vi "PH_Sixpack.panel.vi"(0 "object ref":refnum<vi>, 5 "error in (no error)":errorcluster) -> (19 "error out":errorcluster)   [LabVIEW 2014, in "PH_Sixpack.lvlib"]
doc: "By this VI a hardware switch can be monitored and switched. \n\nThe indicators \"FALSE\", \"TRUE\" and \"SWITCH STATE\" show the value of the Beckhoff-Tag: blue indicates bad tag status reference problems, darkgreen false and lightgreen true. If everything is working fine, \"FALSE\" and \"SWITCH STATE\" should show the same value, while \"TRUE\" has the opposite value. The caption of the sensors for \"FALSE\" and \"TRUE\" are taken out of the database. In case of only one or no sensor these GUI elements are not shown at all.\n\nThe oval button switches. It should be in the same state as the \"SWITCH STATE\" indicator. \n\n\"Delete Instance\" disconnects and removes the instance from the PCS.\n\n\nLicense Agreement for this software:\n\nCopyright (C)\nGesellschaft für Schwerionenforschung, GSI\nPlanckstr. 1\n64291 Darmstadt\nGermany\n\nContact: D.Beck@gsi.de \n\nThis program is free software; you can redistribute it and/or modify it under the terms of the GNU General Public License as published by the Free Software Foundation; either version 2 of the license, or (at your option) any later version.\n\nThis program is distributed in the hope that it will be useful, but WITHOUT ANYW ARRANTY; without even the implied warranty of MERCHANTABILITY or FITNESS FOR A PARTICULAR PURPOSE. See the GNU General License for more details (http://www.gnu.org).\n\nGesellschaft für Schwerionenforschung, GSI\nPlanckstr. 1, 64291 Darmstadt, Germany\nFor all questions and ideas contact: M.Richter@gsi.de, H.Brand@gsi.de or D.Beck@gsi.de.\nLast update: 18-DEC-2002"
uses:
  PH_Sixpack.lvlib
  PH_Stepmotor_BaseClass/PH_Stepmotor_BaseClass.Axis Settings.ctl
  PH_Stepmotor_BaseClass/PH_Stepmotor_BaseClass.Motor Type.ctl
  PH_Stepmotor_BaseClass/PH_Stepmotor_BaseClass.Axis Information.ctl
  PH_Stepmotor_BaseClass/PH_Stepmotor_BaseClass.Axis Activity.ctl
  PH_Sixpack.Status.ctl
  PH_Sixpack.Axis Cluster.ctl
  PH_Sixpack.Axis Configuration.ctl
  instr.lib/SixPack/PackDLL/VmaxAmax.ctl
  instr.lib/SixPack/PackDLL/PeakCurrent.ctl
  instr.lib/SixPack/PackDLL/VStartVmin.ctl
  instr.lib/SixPack/PackDLL/Ref Search Parameter.ctl
  instr.lib/SixPack/PackDLL/Stopswitch Limits.ctl
  instr.lib/SixPack/PackDLL/Motor Parameter.ctl
  instr.lib/SixPack/PackDLL/MotorParameter_P5.ctl
  instr.lib/SixPack/PackDLL/MotorParameter_P6.ctl
  instr.lib/SixPack/PackDLL/Current Control.ctl
  instr.lib/SixPack/PackDLL/Current.ctl
  PH_Sixpack.Input.ctl
  PH_Stepmotor_BaseClass/PH_Stepmotor_BaseClass.GUI Refs.ctl
  CSCore/CSObj/CSObj.lvlib
  PH_Common/PH_Common.lvlib
  PH_Stepmotor_BaseClass/PH_Stepmotor_BaseClass.lvlib
  PH_Class/PH_Class.lvlib
  instr.lib/SixPack/Sixpack - Driver.lvlib
panel:
  out "PeriodicInterval [ms]":i32=-1
  out "Inputs":T1[](array[typedef])
  out "Axes Configuration (Sixpack)":T2[](array[typedef]) {"Config"."Axis Parameter"."Poslimit (6400)" step=1; "Config"."Ref Search Parameter"."DebouncingTime (22ms)" format="%.0x"; "Config"."I max (50%)" min=0.0 max=100.0}
  out "Axes PSDB Infos":T14(array[cluster])
  out "Axis to do a RefSearch":i32=-1
  out "Status":T15
  out "Firmwareversion":dbl=-1.0
  out "Serial Number":dbl=-1.0
  out "Information":T16={"SixPack ID(0)"=0, "BaudRate(19200)"=19200, "COM Port"=enum."COM1", "HANDLE"=0}
  out "Device Error":errorcluster
  out "Axes Configuration (Base Class)":T21(array[cluster])
  in  "Stop":bool caption="SetZero"
  out "PSDB Status":u32(colorbox)=6618880 caption="PSDB"
  in  "Exit":bool
  in  "Delete":bool
  # "PCS"
  # "3.40"
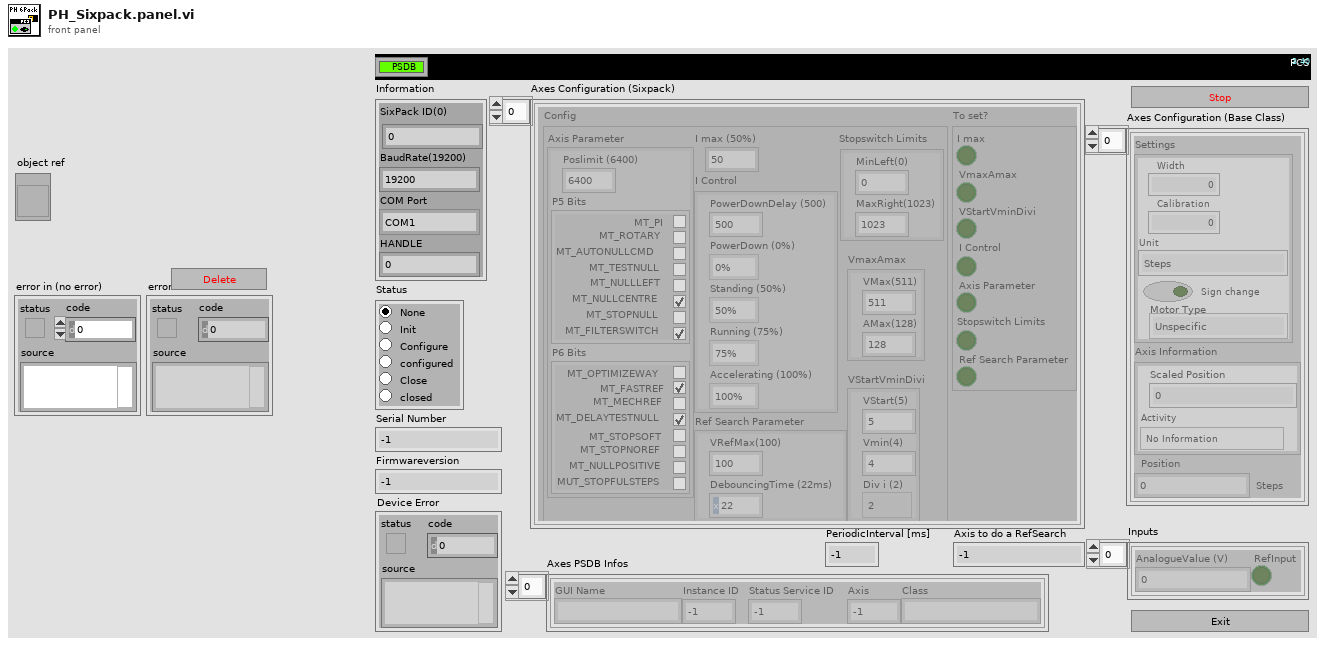
[diagram p1: front panel]
types:
  T1 = typedef "PH_Sixpack.lvlib/PH_Sixpack.Input.ctl" = cluster{"AnalogueValue (V)":dbl, "RefInput":bool}
  T2 = typedef "PH_Sixpack.lvlib/PH_Sixpack.Axis Cluster.ctl" = cluster{"Config":T3, "To set?":cluster{"VmaxAmax":bool, "I max":bool, "VStartVminDivi":bool, "Ref Search Parameter":bool, "Stopswitch Limits":bool, "Axis Parameter":bool, "I Control":bool}}
  T3 = typedef "PH_Sixpack.lvlib/PH_Sixpack.Axis Configuration.ctl" = cluster{"VmaxAmax":T4, "I max (50%)":T5, "VStartVminDivi":T6, "Ref Search Parameter":T7, "Stopswitch Limits":T8, "Axis Parameter":T9, "I Control":T12}
  T4 = typedef "Sixpack - Driver.lvlib/VmaxAmax.ctl" = cluster{"VMax(511)":u16, "AMax(128)":u16}
  T5 = typedef "Sixpack - Driver.lvlib/PeakCurrent.ctl" = dbl
  T6 = typedef "Sixpack - Driver.lvlib/VStartVmin.ctl" = cluster{"VStart(5)":u16, "Vmin(4)":u16, "Div i (2)":enum8{"0", "1", "2", "3"}}
  T7 = typedef "Sixpack - Driver.lvlib/Ref Search Parameter.ctl" = cluster{"VRefMax(100)":u16, "DebouncingTime (22ms)":u8}
  T8 = typedef "Sixpack - Driver.lvlib/Stopswitch Limits.ctl" = cluster{"MinLeft(0)":u16, "MaxRight(1023)":u16}
  T9 = typedef "Sixpack - Driver.lvlib/Motor Parameter.ctl" = cluster{"Poslimit (6400)":u32, "P5 Bits":T10, "P6 Bits":T11}
  T10 = typedef "Sixpack - Driver.lvlib/MotorParameter_P5.ctl" = cluster{"MT_PI":bool, "MT_ROTARY":bool, "MT_AUTONULLCMD":bool, "MT_TESTNULL":bool, "MT_NULLLEFT":bool, "MT_NULLCENTRE":bool, "MT_STOPNULL":bool, "MT_FILTERSWITCH":bool}
  T11 = typedef "Sixpack - Driver.lvlib/MotorParameter_P6.ctl" = cluster{"MT_OPTIMIZEWAY":bool, "MT_FASTREF":bool, "MT_MECHREF":bool, "MT_DELAYTESTNULL":bool, "MT_STOPSOFT":bool, "MT_STOPNOREF":bool, "MT_NULLPOSITIVE":bool, "MUT_STOPFULSTEPS":bool}
  T12 = typedef "Sixpack - Driver.lvlib/Current Control.ctl" = cluster{"PowerDownDelay (500)":u16, "PowerDown (0%)":T13, "Standing (50%)":T13, "Running (75%)":T13, "Accelerating (100%)":T13}
  T13 = typedef "Sixpack - Driver.lvlib/Current.ctl" = enum8{"100%", "75%", "50%", "38%", "25%", "19%", "13%", "9%", "0%"}
  T14 = cluster{"GUI Name":string, "Instance ID":i32, "Status Service ID":i32, "Axis":i32, "Class":string}[]
  T15 = typedef "PH_Sixpack.lvlib/PH_Sixpack.Status.ctl" = enum32{"None", "Init", "Configure", "configured", "Close", "closed"}
  T16 = cluster{"SixPack ID(0)":u16, "BaudRate(19200)":u16, "COM Port":enum32{"COM1", "COM2", "COM3", "COM4", "COM5", "COM6", "COM7", "COM8", "COM9"}, "HANDLE":i32}
  T17 = typedef "PH_Stepmotor_BaseClass.lvlib/PH_Stepmotor_BaseClass.Axis Settings.ctl" = cluster{"Sign change":bool, "Width":dbl, "Calibration":dbl, "Unit":string, "Motor Type":T18, "Unit Width":string, "Unit CF":string}
  T18 = typedef "PH_Stepmotor_BaseClass.lvlib/PH_Stepmotor_BaseClass.Motor Type.ctl" = enum16{"Unspecific", "OWIS 49.120.2633", "OWIS 49.060.1033", "OWIS 43.040.2558", "Diamond Motion 2200 series", "OWIS 49.120.266B.MV6", "Calorimeter", "Linear Stage 1", "MICOS VT-80", "MICOS VT-80 S", "Standa Rotstage nt0.95A", "PUF RA 320.200", "PUF RA 800.200", "PUF RA 800.400", "PUF RA 400.50", "1324.nn.800.50", "1324.n9c.800.50", "1324.nn.320.200", "1324.nn.400.200", "1324.nn.800.200", "1324.nn.400.50", "1324.8c9c.800.50", "1324.8c9c.400.200"}
  T19 = typedef "PH_Stepmotor_BaseClass.lvlib/PH_Stepmotor_BaseClass.Axis Information.ctl" = cluster{"Scaled Position":dbl, "Activity":T20}
  T20 = typedef "PH_Stepmotor_BaseClass.lvlib/PH_Stepmotor_BaseClass.Axis Activity.ctl" = enum16{"No Information", "stopped", "running", "Failure", "Alarm", "stopped at backward ES", "stopped at foreward ES"}
  T21 = cluster{"Settings":T17, "Axis Information":T19, "Position":i32}[]
  T22 = typedef "PH_Stepmotor_BaseClass.lvlib/PH_Stepmotor_BaseClass.GUI Refs.ctl" = cluster{"Axes Configuration":refnum<vi>, "Device Error":refnum<vi>, "Axes PSDB Infos":refnum<vi>}
  T23 = cluster{"Stepmotor Base Class ":T22, "PSDB Status":refnum<vi>}
  T24 = typedef "PH_Sixpack.lvlib/PH_Sixpack.i attribute.ctl" = cluster{"Information":cluster{"SixPack ID(0)":u16, "BaudRate(19200)":u16, "COM Port":enum32{"COM1", "COM2", "COM3", "COM4", "COM5", "COM6", "COM7", "COM8", "COM9"}, "HANDLE":i32}, "Serial Number":dbl, "Firmwareversion":dbl, "Axes":T2[], "Status":T15, "Axis to do a RefSearch":i32, "GUI Refs":cluster{"Information":refnum<vi>, "Serial Number":refnum<vi>, "Firmwareversion":refnum<vi>, "Status":refnum<vi>, "Axis to do a RefSearch":refnum<vi>, "Axes Configuration (Sixpack)":refnum<vi>, "Inputs":refnum<vi>, "PeriodicInterval [ms]":refnum<vi>}, "Constructor finished":bool, "Ignore Error":bool}
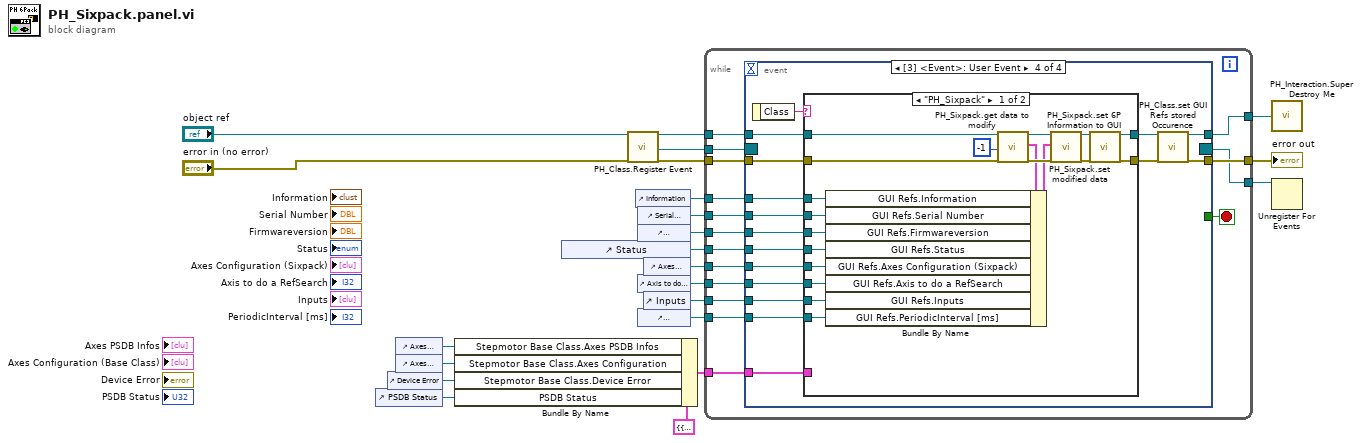
[diagram p0: block diagram]
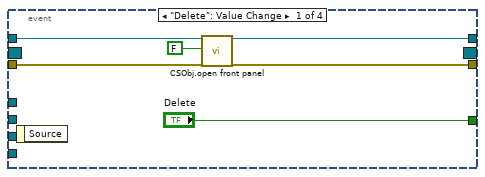
[diagram p2: hidden frame]
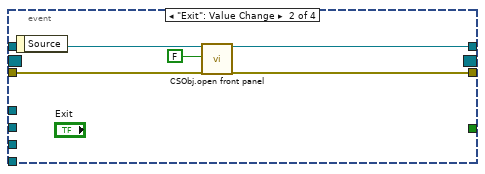
[diagram p3: hidden frame]
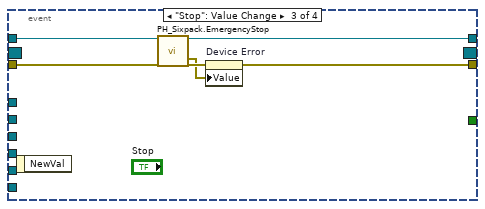
[diagram p4: hidden frame]
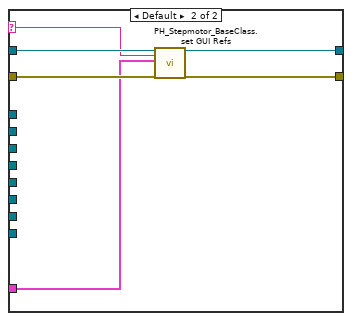
[diagram p5: hidden frame]
diagram:
  n1 = control-ref of="PSDB Status"() -> (w12:refnum<vi>)
  n2 = control-ref of="Device Error"() -> (w13:refnum<vi>)
  n3 = control-ref of="Axes PSDB Infos"() -> (w15:refnum<vi>)
  n4 = control-ref of="Axes Configuration (Base Class)"() -> (w14:refnum<vi>)
  n5 = Bundle By Name(cluster=T23 {"Stepmotor Base Class "={"Axes Configuration"=refnum, "Device Error"=refnum, "Axes PSDB Infos"=refnum}, "PSDB Status"=refnum} ("GUI Refs"), "Stepmotor Base Class.Axes PSDB Infos"=w15, "Stepmotor Base Class.Axes Configuration"=w14, "Stepmotor Base Class.Device Error"=w13, "PSDB Status"=w12) -> (w16:T23)
  n6 = control-ref of="Status"() -> (w8:refnum<vi>)
  n7 = call "PH_Class.Register Event.vi"("i ref in"="object ref", "error in (no error)"="error in (no error)") -> ("i ref out"=w20:refnum<vi>, "Event Registration Refnum"=w18:refnum<event-registration>, "error out"=w19:errorcluster)  [unwired: 15 in]
  n8 = control-ref of="Information"() -> (w11:refnum<vi>)
  n9 = control-ref of="Serial Number"() -> (w10:refnum<vi>)
  n10 = control-ref of="Firmwareversion"() -> (w9:refnum<vi>)
  n11 = control-ref of="Axis to do a RefSearch"() -> (w6:refnum<vi>)
  n12 = control-ref of="PeriodicInterval [ms]"() -> (w4:refnum<vi>)
  n13 = control-ref of="Axes Configuration (Sixpack)"() -> (w7:refnum<vi>)
  n14 = control-ref of="Inputs"() -> (w5:refnum<vi>)
  n15 = while {
    tunnel: w20 -> [w35]
    tunnel: [w34] -> w22
    tunnel: w19 -> [w37]
    tunnel: [w36] -> w21
    tunnel: w18 -> [w33]
    tunnel: w16 -> [w32]
    tunnel: w11 -> [w31]
    tunnel: w10 -> [w30]
    tunnel: w9 -> [w29]
    tunnel: w8 -> [w28]
    tunnel: w7 -> [w27]
    tunnel: w6 -> [w26]
    tunnel: w5 -> [w25]
    tunnel: w4 -> [w24]
    tunnel: [w23] -> w1
    stop <- w38 stop-if-true
    n16 = event shown="[3] <Event>: User Event" {
      selector: w33 -> [_ _ _ _]
      dyn-events: [_ _ _ _] -> w23
      timeout: _ -> [_ _ _ _]
      tunnel: ["Delete" _ _ _] -> w38
      tunnel: w35 -> [w40 w48 w54 w71]
      tunnel: w37 -> [w39 w47 w55 w70]
      tunnel: [w42 w46 w51 w58] -> w36
      tunnel: [w41 w45 w53 w56] -> w34
      tunnel: w32 -> [_ _ _ w68]
      tunnel: w31 -> [_ _ _ w66]
      tunnel: w30 -> [_ _ _ w65]
      tunnel: w29 -> [_ _ _ w64]
      tunnel: w28 -> [_ _ _ w63]
      tunnel: w27 -> [_ _ _ w62]
      tunnel: w26 -> [_ _ _ w61]
      tunnel: w25 -> [_ _ _ w60]
      tunnel: w24 -> [_ _ _ w59]
      event "Delete": Value Change {
        n17 = event-data() -> ()  [unwired: 1 in, 1 out]
        n18 = call "CSObj.open front panel.vi"("i ref in"=w40, "frontPanelOpen"=FALSE ("front panel open"), "error in (no error)"=w39) -> ("i ref out"=w41:refnum<vi>, "error out"=w42:errorcluster)  [unwired: 15 in]
      }
      event "Exit": Value Change {
        n19 = event-data() -> ()  [unwired: 1 in, 1 out]
        n20 = call "CSObj.open front panel.vi"("i ref in"=w48, "frontPanelOpen"=FALSE ("front panel open"), "error in (no error)"=w47) -> ("i ref out"=w45:refnum<vi>, "error out"=w46:errorcluster)  [unwired: 15 in]
      }
      event "Stop": Value Change {
        n21 = event-data() -> ()  [unwired: 1 in, 1 out]
        n22 = call "PH_Sixpack.EmergencyStop.vi"("i ref in"=w54, "error in"=w55) -> ("i ref out"=w53:refnum<vi>, "Device Error out"=w50:errorcluster, "error out"=w52:errorcluster)  [unwired: 15 in]
        n23 = property on="Device Error" class="Clust (strict)"(error in=w52, "Value"=w50) -> (error out=w51:errorcluster)  [unwired: 1 in, 1 out]
      }
      event User Event {
        n24 = event-data() -> ("Class"=w67:string)  [unwired: 1 in]
        n25 = case shown="\"PH_Sixpack\"" w67 {
          selector: w67 -> [_ w91]
          tunnel: w71 -> [w83 w96]
          tunnel: w70 -> [w82 w95]
          tunnel: [w73 w94] -> w57
          tunnel: [w72 w93] -> w69
          tunnel: w68 -> [_ w92]
          tunnel: w66 -> [w81 _]
          tunnel: w65 -> [w80 _]
          tunnel: w64 -> [w79 _]
          tunnel: w63 -> [w78 _]
          tunnel: w62 -> [w77 _]
          tunnel: w61 -> [w76 _]
          tunnel: w60 -> [w75 _]
          tunnel: w59 -> [w74 _]
          frame "PH_Sixpack" {
            n26 = call "PH_Sixpack.get data to modify.vi"("i ref in"=w83, "ms timeout (10000)"=-1, "error in (no error)"=w82) -> ("i ref out"=w89:refnum<vi>, "i attribute"=w87:T24, "error out"=w90:errorcluster)  [unwired: 13 in, 1 out]
            n27 = Bundle By Name(cluster=w87, "GUI Refs.Information"=w81, "GUI Refs.Serial Number"=w80, "GUI Refs.Firmwareversion"=w79, "GUI Refs.Status"=w78, "GUI Refs.Axes Configuration (Sixpack)"=w77, "GUI Refs.Axis to do a RefSearch"=w76, "GUI Refs.Inputs"=w75, "GUI Refs.PeriodicInterval [ms]"=w74) -> (w86:T24)
            n28 = call "PH_Sixpack.set modified data.vi"("i ref in"=w89, "i attribute"=w86, "error in (no error)"=w90) -> ("i ref out"=w85:refnum<vi>, "error out"=w84:errorcluster)  [unwired: 15 in]
            n29 = call "PH_Sixpack.set 6P Information to GUI.vi"("VI in"=w85, "error in (no error)"=w84) -> ("VI out"=w73:refnum<vi>, "error out"=w72:errorcluster)  [unwired: 16 in]
          }
          frame Default {
            n30 = call "PH_Stepmotor_BaseClass.set GUI Refs.vi"("i ref in"=w96, "Class"=w91, "GUI Refs"=w92, "error in"=w95) -> ("i ref out"=w94:refnum<vi>, "error out"=w93:errorcluster)  [unwired: 14 in]
          }
        }
        n31 = call "PH_Class.set GUI Refs stored Occurence.vi"("i ref in"=w57, "error in (no error)"=w69) -> ("i ref out"=w56:refnum<vi>, "error out"=w58:errorcluster)  [unwired: 16 in]
      }
    }
  }
  "error out" <- w21
  n32 = call "PH_Interaction.Super Destroy Me.vi"("i ref out"=w22) -> ()
  n33 = Unregister For Events(event registration refnum=w1) -> ()  [unwired: 1 in, 1 out]
